vi "linkToUI_equipos.vi"(8 "error in (no error)":errorcluster, 9 "Pane VI":string="AjustePrevio1.vi", 10 "subPanel":refnum<vi>, 11 "Equipo in":refnum<class "Equipo.lvclass">) -> (0 "error out":errorcluster, 3 "Equipo out":refnum<class "Equipo.lvclass">)   [LabVIEW 2019, in "Equipo.lvclass"]
uses:
  Equipo.lvclass
  User Interface/UI.lvclass
  PanelFactory/PanelFactory.lvclass
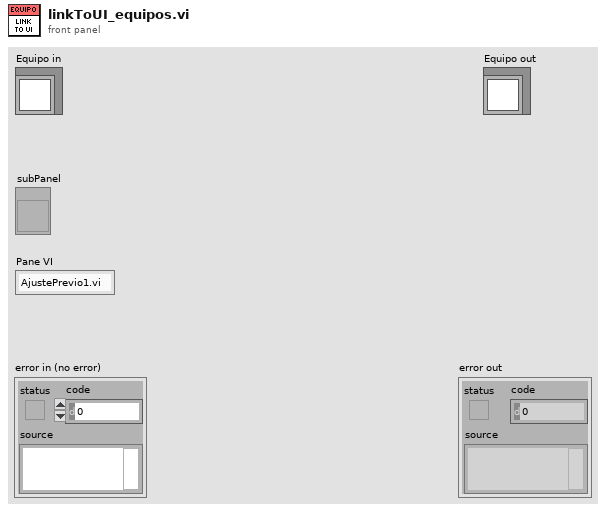
[diagram p1: front panel]
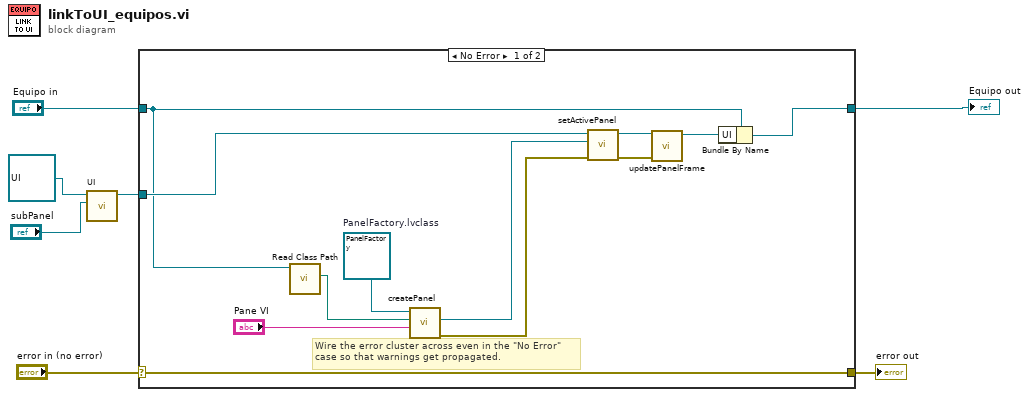
[diagram p0: block diagram]
diagram:
  n1 = call "UI.vi"("subPanel"="subPanel", "UI in"=refnum<class "UI.lvclass"> refnum ("UI.lvclass")) -> ("UI out"=w4:refnum<class "UI.lvclass">)  [unwired: 8 in, 1 out]
  n2 = case shown="No Error" "error in (no error)" {
    selector: "error in (no error)" -> [w19 w21]
    tunnel: [w19 w21] -> w6
    tunnel: "Equipo in" -> [w8 w20]
    tunnel: w4 -> [w15 _]
    tunnel: [w10 w20] -> w1
    frame No Error {
      w18 = refnum<class "PanelFactory.lvclass"> refnum  # PanelFactory.lvclass
      # "Wire the error cluster across even in the \"No Error\"\ncase so that warnings get propagated."
      n3 = call "Read Class Path.vi"("Pruebas in"=w8) -> ("Path to Class"=w9:path)  [unwired: 8 in, 2 out]
      n4 = call "createPanel.vi"("Pane VI"="Pane VI", "Path"=w9, "PanelFactory in"=w18) -> ("error out"=w16:errorcluster, "Panel out"=w17:refnum<class "Panel.lvclass">)  [unwired: 7 in]
      n5 = call "setActivePanel.vi"("error in (no error)"=w16, "Panel"=w17, "UI in"=w15) -> ("error out"=w13:errorcluster, "UI out"=w14:refnum<class "UI.lvclass">)  [unwired: 7 in]
      n6 = call "updatePanelFrame.vi"("error in (no error)"=w13, "UI in"=w14) -> ("UI out"=w12:refnum<class "UI.lvclass">)  [unwired: 8 in, 1 out]
      n7 = Bundle By Name(cluster=w8, "UI"=w12) -> (w10:refnum<class "Equipo.lvclass">)
    }
    frame Error {
    }
  }
  "error out" <- w6
  "Equipo out" <- w1
